vi "Test_monitorCommand_fault.vi"(8 "error in (no error)":errorcluster, 11 "command_fault_Ctl":T1) -> (0 "error out":errorcluster, 2 "function return":i32, 3 "command_fault_Ctl out":T1)   [LabVIEW 2016, in "SALLV_Test.lvlib"]
doc: "int Test_shm_monitorCommand_faultLV(Test_command_faultLV *command_fault_Ctl );"
uses:
  SALLV_Test.lvlib
  DataTypes/command_fault.ctl
  SALLV_Test.so
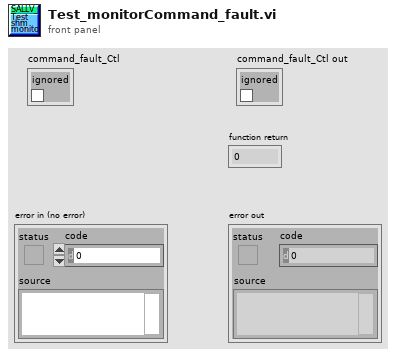
[diagram p1: front panel]
types:
  T1 = typedef "SALLV_Test.lvlib/command_fault.ctl" = cluster{"ignored":bool}
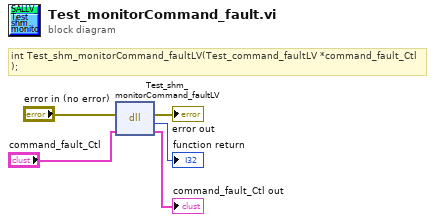
[diagram p0: block diagram]
diagram:
  # "int Test_shm_monitorCommand_faultLV(Test_command_faultLV *command_fault_Ctl );"
  n1 = dll-call lib="home/ccontaxis/Code/SALLV_Test/SALLV_Test.*" fn="Test_shm_monitorCommand_faultLV"(error in="error in (no error)", "command_fault_Ctl"="command_fault_Ctl") -> (error out=→"error out":errorcluster, →"function return":i32, "command_fault_Ctl"=→"command_fault_Ctl out":T1)  [unwired: 2 in, 1 out]
